vi "Noise Processing.vi"() -> ()   [LabVIEW 2017]
panel:
  out "Filtered Signal":dbl
  in  "Waveform":waveform(dbl)
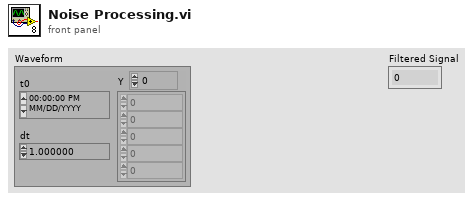
[diagram p1: front panel]
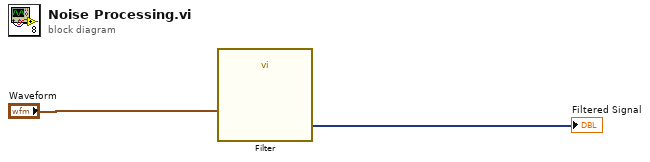
[diagram p0: block diagram]
diagram:
  n1 = call "Filter"("Signal"="Waveform") -> ("Filtered Signal"=→"Filtered Signal":dynamicdata)  [unwired: 9 in, 1 out]
